vi "DriveForDistance.vi"() -> ()   [LabVIEW 2017]
uses:
  Framework/Robot Global Data.vi
panel:
  in  "Distance":dbl
  in  "Speed":dbl
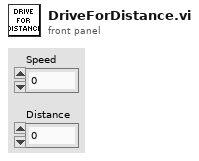
[diagram p1: front panel]
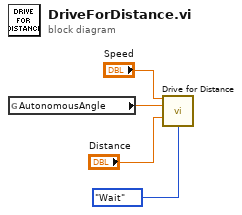
[diagram p0: block diagram]
diagram:
  n1 = global read "Robot Global Data.vi" "AutonomousAngle"() -> (w2:dbl)
  n2 = call "Drive for Distance.vi"("Speed"="Speed", "StartAngle"=w2, "Distance (inch)"="Distance", "Synchronication"=enum16{"Start", "Wait"}."Wait") -> ()  [unwired: 11 in, 1 out]
